vi "Poly App Configuraton Extractor API.vi"(8 "error constant":errorcluster, 11 "General Config DVR In":refnum<data-value>) -> (0 "error out":errorcluster, 3 "Application Configuration":T1)   [LabVIEW 2019, in "Architecture.lvlib"]
doc: "This method extracts is a Poliphormic method used to read each module configuration."
uses:
  Architecture.lvlib
  Typedefs/Application Configuration.ctl
  Modules/Module Template/Typedefs/Config.ctl
  Modules/Module Template/Module Template.lvlib
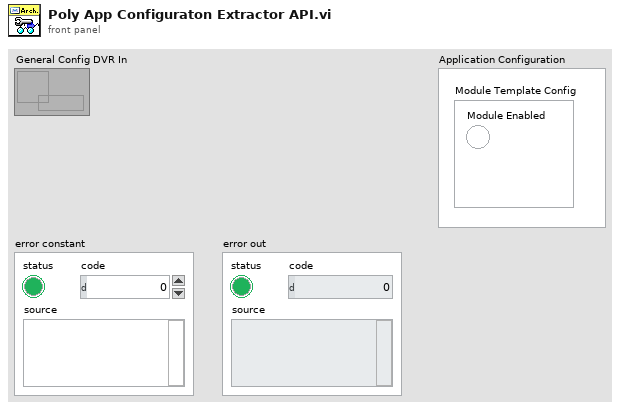
[diagram p1: front panel]
types:
  T1 = typedef "Architecture.lvlib/Application Configuration.ctl" = cluster{"Module Template Config":T2}
  T2 = typedef "Architecture.lvlib/Module Template.lvlib/Config.ctl" = cluster{"Module Enabled":bool}
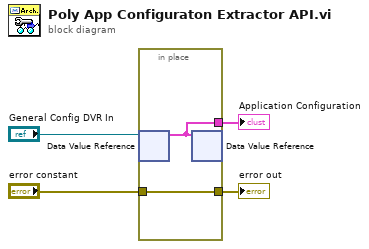
[diagram p0: block diagram]
diagram:
  n1 = in-place {
    in-place-border: [w6] -> w1
    in-place-border: "error constant" -> [w5]
    in-place-border: [w5] -> w2
    n2 = in-place-dvr #1("General Config DVR In") -> (w6:T1)  [unwired: 1 out]
    n3 = in-place-dvr #1(w6) -> ()  [unwired: 2 out]
  }
  "error out" <- w2
  "Application Configuration" <- w1
